vi "Launch Topic.vi"(7 "Include Initial Value? (F)":bool, 9 "Type":variant, 10 "Datum Name":string, 11 "Mediator in":refnum<class "Mediator.lvclass">) -> (0 "error out":errorcluster, 2 "New Topic Enqueuer":refnum<class "Message Enqueuer.lvclass">, 3 "Mediator out":refnum<class "Mediator.lvclass">)   [LabVIEW 2015, in "Mediator.lvlib" / "Mediator.lvclass"]
uses:
  Mediator.lvclass
  <vilib>/ActorFramework/Message Enqueuer/Message Enqueuer.lvclass
  Mediator.lvclass/Mediator.ctl
  SubscriptionPolicy/ValueChangeSubscription/ValueChangeSubscription.lvclass/ValueChangeSubscription.ctl
  Topic Messages/Add Topic Subscriber Msg/Add Topic Subscriber Msg.lvclass/Add Topic Subscriber Msg.ctl
  <vilib>/ActorFramework/Message Enqueuer/Message Enqueuer.lvclass/Message Enqueuer.ctl
  <vilib>/ActorFramework/Message Enqueuer/Enqueue.vi
  <vilib>/ActorFramework/Message Priority Queue/Priority Enqueue.vi
  SubscriptionPolicy/ValueChangeSubscription/ValueChangeSubscription.lvclass
  Topic Messages/Add Topic Subscriber Msg/Add Topic Subscriber Msg.lvclass
  Topic/Topic.lvclass
  <vilib>/ActorFramework/Actor/Actor.lvclass
  TopicLookupTable/TopicLookupTable.lvclass
  IMediator/SubscriptionRequest/SubscriptionRequest.lvclass
  IMediator/ISubscriptionPolicy/ISubscriptionPolicy.lvclass
  IObserver/ActorDataBinding/ActorDataBinding.lvclass
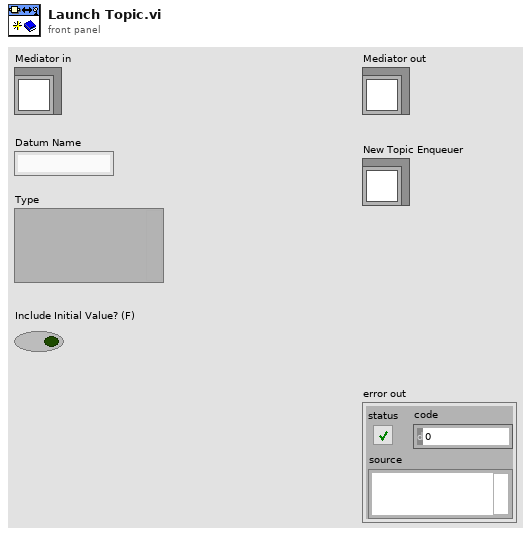
[diagram p1: front panel]
types:
  T1 = typedef "IMediator.lvlib/ISubscriptionPolicy.lvclass/ISubscriptionPolicy Reference.ctl" = refnum<data-value>
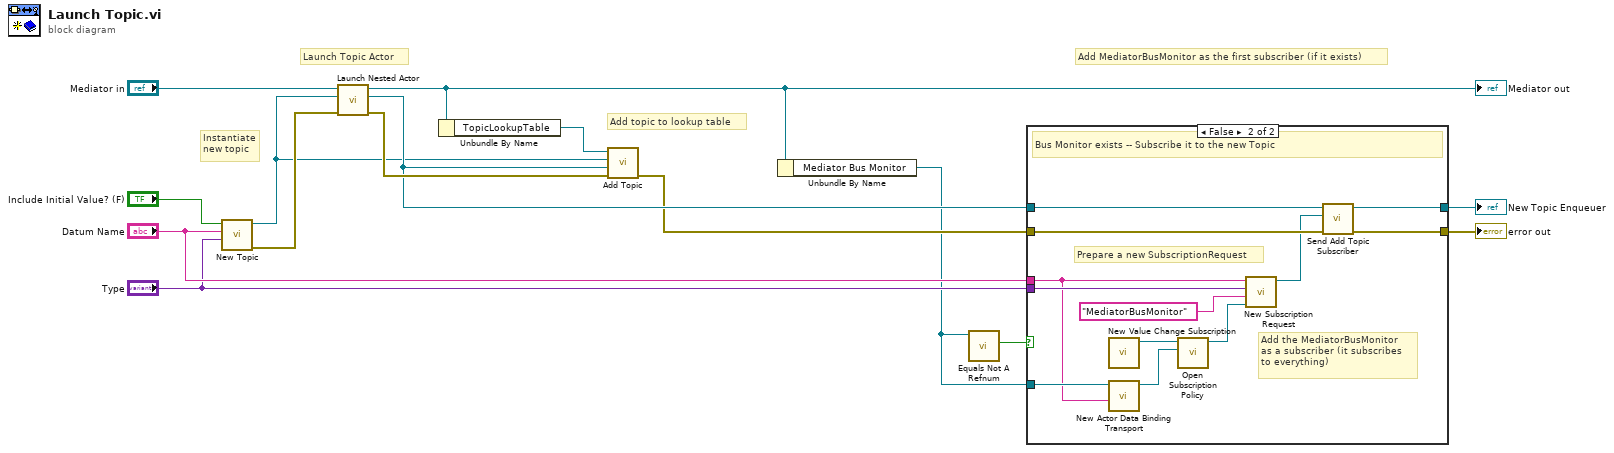
[diagram p0: block diagram]
diagram:
  # "Add MediatorBusMonitor as the first subscriber (if it exists)"
  # "Launch Topic Actor"
  # "Add topic to lookup table"
  # "Instantiate\nnew topic"
  n1 = call "New Topic.vi"("New Topic Data"="Type", "Name"="Datum Name", "Use Type Input As Initial Value?"="Include Initial Value? (F)") -> ("error out"=w9:errorcluster, "Topic out"=w8:refnum<class "Topic.lvclass">)  [unwired: 7 in]
  n2 = call <vilib>:"Launch Nested Actor.vi"("error in (no error)"=w9, "Nested Actor"=w8, "Caller Actor in"="Mediator in") -> ("error out"=w12:errorcluster, "Nested Actor's Enqueuer"=w10:refnum<class "Message Enqueuer.lvclass">, "Caller Actor out"=w4:refnum<class "Mediator.lvclass">)  [unwired: 6 in]
  "Mediator out" <- w4
  n3 = Unbundle By Name(w4) -> ("TopicLookupTable"=w7:refnum<data-value>)
  n4 = call "Add Topic.vi"("error in (no error)"=w12, "Topic Enqueuer"=w10, "Topic Object"=w8, "TopicLookupTable"=w7) -> ("error out"=w6:errorcluster)  [unwired: 5 in, 2 out]
  n5 = Unbundle By Name(w4) -> ("Mediator Bus Monitor"=w2:refnum<class "Message Enqueuer.lvclass">)
  n6 = call <vilib>:"Equals Not A Refnum.vi"("Message Enqueuer"=w2) -> ("Not a refnum?"=w3:bool)  [unwired: 10 in]
  n7 = case shown="False" w3 {
    tunnel: "Datum Name" -> [_ w18]
    tunnel: "Type" -> [_ w25]
    tunnel: [w17 w24] -> w11
    tunnel: w10 -> [w17 w23]
    tunnel: w6 -> [w16 w22]
    tunnel: [w16 w21] -> w5
    tunnel: w2 -> [_ w19]
    frame True {
      # "Actor queue = Not a refnum -- Bus Monitor does not exist"
    }
    frame False {
      # "Prepare a new SubscriptionRequest"
      # "Add the MediatorBusMonitor\nas a subscriber (it subscribes\nto everything)"
      # "Bus Monitor exists -- Subscribe it to the new Topic"
      n8 = call "New Value Change Subscription.vi"() -> ("ValueChangeSubscription Out"=w28:refnum<class "ValueChangeSubscription.lvclass">)  [unwired: 11 in]
      n9 = call "New Actor Data Binding Transport.vi"("Datum Return Name"=w18, "IObserver"=w19) -> ("ActorDataBinding out"=w29:refnum<class "ActorDataBinding.lvclass">)  [unwired: 8 in, 1 out]
      n10 = call "Open Subscription Policy.vi"("Transport"=w29, "SubscriptionPolicy"=w28) -> ("Subscription Policy"=w27:T1)  [unwired: 8 in, 1 out]
      n11 = call "New Subscription Request.vi"("Subscription Policy"=w27, "Unique Subscriber ID"="MediatorBusMonitor", "Type"=w25, "Datum Name"=w18) -> ("SubscriptionRequest"=w20:refnum<class "SubscriptionRequest.lvclass">)  [unwired: 7 in]
      n12 = call "Send Add Topic Subscriber.vi"("error in (no error)"=w22, "Subscription Request"=w20, "Message Enqueuer"=w23) -> ("error out"=w21:errorcluster, "Message Enqueuer out"=w24:refnum<class "Message Enqueuer.lvclass">)  [unwired: 7 in]
    }
  }
  "error out" <- w5
  "New Topic Enqueuer" <- w11
